vi "CB State Space.vi"(6 "dt":dbl=-1.0, 8 "D":T2, 9 "C":T2, 10 "B":T2, 11 "A":T2) -> (0 "error out":errorcluster, 3 "State Space Model":T1)   [LabVIEW 2020]
uses:
  <vilib>/Analysis/Matrix/Datatypes/RealMatrix.ctl
  CB State Space.ctl
  <vilib>/Analysis/Matrix/NI_Matrix.lvlib
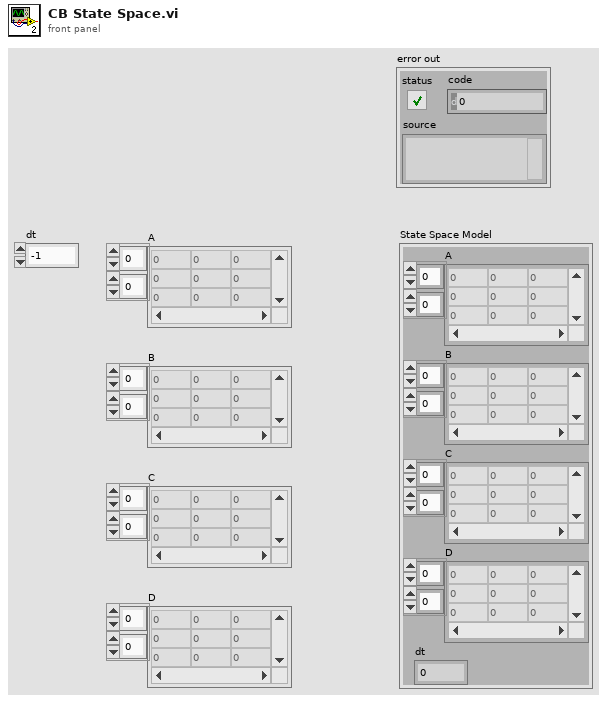
[diagram p1: front panel]
types:
  T1 = typedef "CB State Space.ctl" = cluster{"A":T2, "B":T2, "C":T2, "D":T2, "dt":dbl}
  T2 = typedef "NI_Matrix.lvlib/RealMatrix.ctl" = dbl[][]
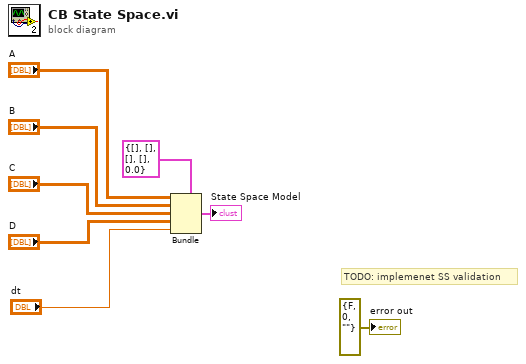
[diagram p0: block diagram]
diagram:
  # "TODO: implemenet SS validation"
  n1 = Bundle(cluster=T1 {"A"=[], "B"=[], "C"=[], "D"=[], "dt"=0.0} ("output cluster"), "A"="A", "B"="B", "C"="C", "D"="D", "dt"="dt") -> (→"State Space Model":T1)
  "error out" <- errorcluster {"status"=FALSE, "code"=0, "source"=""} ("error constant")
